vi "SmartSEM Remote API goto min or max FIB probe current.vi"(8 "error in":errorcluster, 9 "Min or Max":string(combo)="Min", 10 "FIB Probe":string(combo), 11 "Api":refnum<k7>(container)) -> (2 "Goto probe":string, 3 "Api out":refnum<k7>)   [LabVIEW 2018]
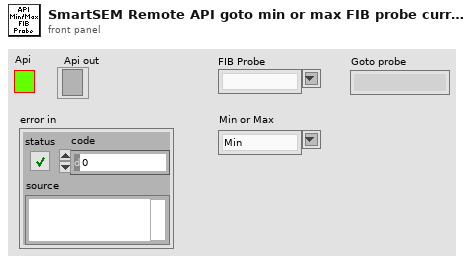
[diagram p1: front panel]
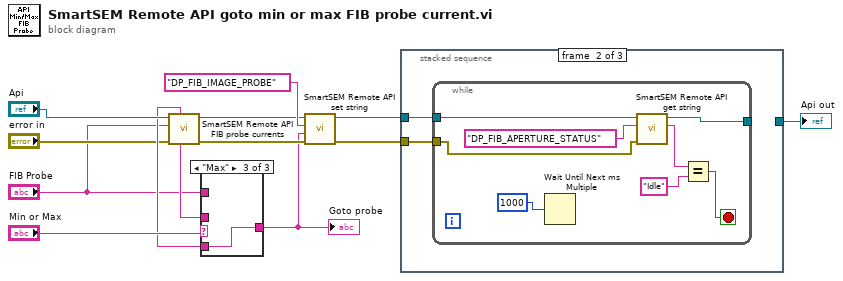
[diagram p0: block diagram]
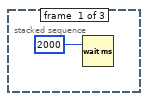
[diagram p2: hidden frame]
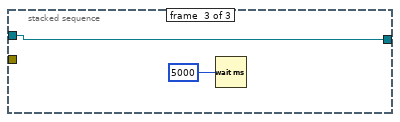
[diagram p3: hidden frame]
diagram:
  n1 = call "SmartSEM Remote API FIB probe currents.vi"("error in"="error in", "FIB Probe"="FIB Probe", "Api"="Api") -> ("error out"=w10:errorcluster, "Api out"=w11:refnum<k7>, "Min probe"=w8:string, "Max probe"=w7:string)  [unwired: 1 in, 4 out]
  n2 = case shown="\"Max\"" "Min or Max" {
    tunnel: w8 -> [_ w15 _]
    tunnel: w7 -> [_ _ w16]
    tunnel: [w14 w15 w16] -> w6
    tunnel: "FIB Probe" -> [w14 _ _]
    frame Default {
    }
    frame "Min" {
    }
    frame "Max" {
    }
  }
  "Goto probe" <- w6
  n3 = call "SmartSEM Remote API set string.vi"("error in"=w10, "vValue"=w6, "lpszParam"="DP_FIB_IMAGE_PROBE", "Api"=w11) -> ("error out"=w1:errorcluster, "Api out"=w2:refnum<k7>)  [unwired: 6 in]
  n4 = stacked-sequence {
    tunnel: w2 -> [_ w19 w28]
    tunnel: [_ _ w28] -> w5
    tunnel: w1 -> [_ w18 _]
    frame #0 {
      n5 = Wait (ms)(milliseconds to wait=u32 2000) -> ()  [unwired: 1 out]
    }
    frame #1 {
      n6 = while {
        tunnel: w19 -> [w24]
        tunnel: [w23] -> _
        tunnel: w18 -> [w22]
        stop <- w25 stop-if-true
        n7 = Wait Until Next ms Multiple(millisecond multiple=u32 1000) -> ()  [unwired: 1 out]
        n8 = call "SmartSEM Remote API get string.vi"("error in"=w22, "lpszParam"="DP_FIB_APERTURE_STATUS", "Api"=w24) -> ("data"=w21:string, "Api out"=w23:refnum<k7>)  [unwired: 6 in, 1 out]
        n9 = Equal?(x=w21, y="Idle" ("lpszParam")) -> (x = y?=w25:bool)
      }
    }
    frame #2 {
      n10 = Wait (ms)(milliseconds to wait=u32 5000) -> ()  [unwired: 1 out]
    }
  }
  "Api out" <- w5
